vi "Numeric Alarm.vi"(10 "Simple Alarm Values":T1={"tag name"="mytag", "HiHi"=90.0, "Hi"=75.0, "Lo"=25.0, "LoLo"=10.0}, 11 "Alarms in":T2(array[cluster])=[{"enable? (F)"=TRUE, "name"="", "alarm type"=enum."HI_HI", "level/change"=0.0, "deadband/time"=1.0, "priority"=500, "ack type"=enum."Each Occurrence", "area"="", "description"="", "log? (T)"=TRUE}, {"enable? (F)"=TRUE, "name"="", "alarm type"=enum."HI", "level/change"=0.0, "deadband/time"=1.0, "priority"=1, "ack type"=enum."Each Occurrence", "area"="", "description"="", "log? (T)"=TRUE}, {"enable? (F)"=TRUE, "name"="", "alarm type"=enum."LO", "level/change"=0.0, "deadband/time"=1.0, "priority"=1, "ack type"=enum."Each Occurrence", "area"="", "description"="", "log? (T)"=TRUE}, {"enable? (F)"=TRUE, "name"="", "alarm type"=enum."LO_LO", "level/change"=0.0, "deadband/time"=1.0, "priority"=500, "ack type"=enum."Each Occurrence", "area"="", "description"="", "log? (T)"=TRUE}]) -> (3 "Alarms out":T2(array[cluster])=[{"enable? (F)"=TRUE, "name"="mytag:HiHi", "alarm type"=enum."HI_HI", "level/change"=90.0, "deadband/time"=1.0, "priority"=500, "ack type"=enum."Each Occurrence", "area"="", "description"="", "log? (T)"=TRUE}, {"enable? (F)"=TRUE, "name"="mytag:Hi", "alarm type"=enum."HI", "level/change"=75.0, "deadband/time"=1.0, "priority"=1, "ack type"=enum."Each Occurrence", "area"="", "description"="", "log? (T)"=TRUE}, {"enable? (F)"=TRUE, "name"="mytag:Lo", "alarm type"=enum."LO", "level/change"=25.0, "deadband/time"=1.0, "priority"=1, "ack type"=enum."Each Occurrence", "area"="", "description"="", "log? (T)"=TRUE}, {"enable? (F)"=TRUE, "name"="mytag:LoLo", "alarm type"=enum."LO_LO", "level/change"=10.0, "deadband/time"=1.0, "priority"=500, "ack type"=enum."Each Occurrence", "area"="", "description"="", "log? (T)"=TRUE}])   [LabVIEW 2018, in "Dynamic Shared Variables.lvlib"]
doc: "Create a numeric alarm configuration with some defaults."
uses:
  Dynamic Shared Variables.lvlib
  Simple Alarm Values Cluster.ctl
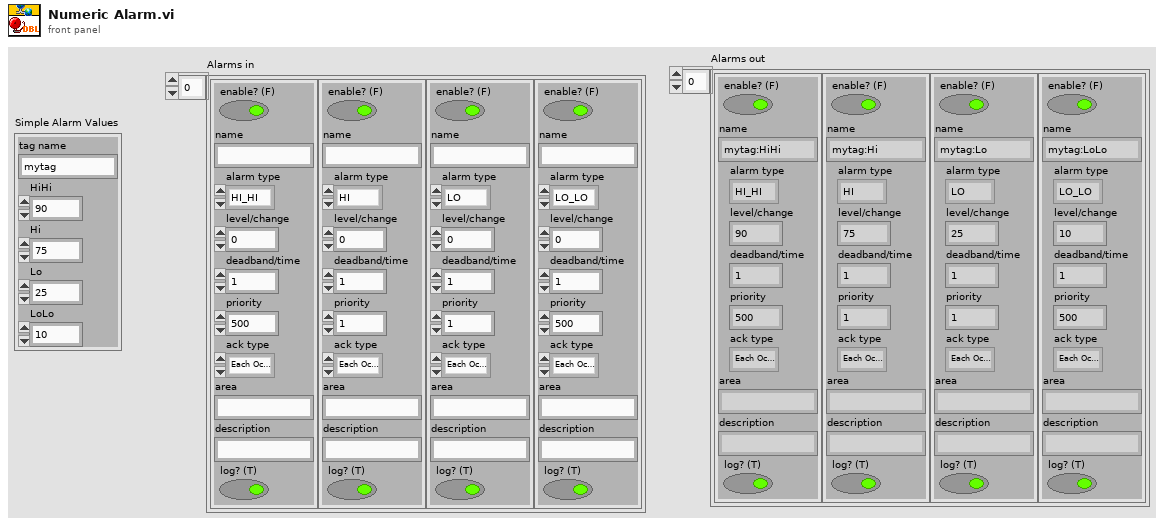
[diagram p1: front panel]
types:
  T1 = typedef "Dynamic Shared Variables.lvlib/Simple Alarm Values Cluster.ctl" = cluster{"tag name":string, "HiHi":dbl, "Hi":dbl, "Lo":dbl, "LoLo":dbl}
  T2 = cluster{"enable? (F)":bool, "name":string, "alarm type":enum16{"HI_HI", "HI", "LO", "LO_LO"}, "level/change":dbl, "deadband/time":dbl, "priority":u32, "ack type":enum16{"Auto", "User", "None", "Each Occurrence"}, "area":string, "description":string, "log? (T)":bool}[]
  T3 = cluster{"enable? (F)":bool, "name":string, "alarm type":enum16{"HI_HI", "HI", "LO", "LO_LO"}, "level/change":dbl, "deadband/time":dbl, "priority":u32, "ack type":enum16{"Auto", "User", "None", "Each Occurrence"}, "area":string, "description":string, "log? (T)":bool}
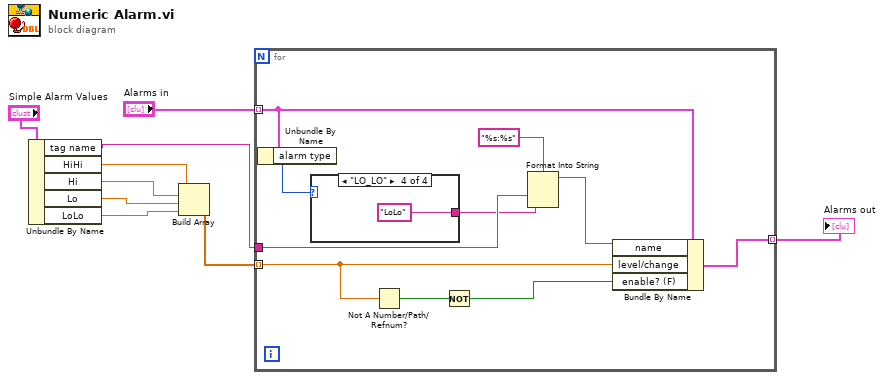
[diagram p0: block diagram]
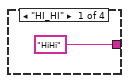
[diagram p2: hidden frame]
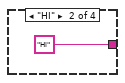
[diagram p3: hidden frame]
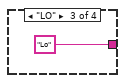
[diagram p4: hidden frame]
diagram:
  n1 = Unbundle By Name("Simple Alarm Values") -> ("tag name"=w5:string, "HiHi"=w4:dbl, "Hi"=w3:dbl, "Lo"=w2:dbl, "LoLo"=w1:dbl)
  n2 = Build Array(w4, w3, w2, w1) -> (w8:dbl[])
  n3 = for {
    tunnel: w5 -> [w15]
    tunnel: "Alarms in" -> [w18] mode=indexing
    tunnel: w8 -> [w12] mode=indexing
    tunnel: [w19] -> w7 mode=indexing
    n4 = Unbundle By Name(w18) -> ("alarm type"=w17:enum16{"HI_HI", "HI", "LO", "LO_LO"})
    n5 = case shown="\"LO_LO\"" w17 {
      tunnel: ["HiHi" "Hi" "Lo" "LoLo"] -> w14
      frame "HI_HI" {
      }
      frame "HI" {
      }
      frame "LO" {
      }
      frame "LO_LO" {
      }
    }
    n6 = Not A Number/Path/Refnum?(number/path/refnum=w12) -> (NaN/Path/Refnum?=w11:bool)
    n7 = Not(x=w11) -> (.not. x?=w10:bool)
    n8 = Format Into String(format string="%s:%s", w15, w14) -> (resulting string=w13:string)  [unwired: 2 in, 1 out]
    n9 = Bundle By Name(cluster=w18, "name"=w13, "level/change"=w12, "enable? (F)"=w10) -> (w19:T3)
  }
  "Alarms out" <- w7
